vi "LWXPS_CPUCoreAndBoardSupplyVoltagesGet.vi"(1 "XPS Reference IN":refnum<k24>, 4 "LabVIEW error IN":errorcluster) -> (8 "XPS Reference OUT":refnum<k24>, 9 "LabVIEW error OUT":errorcluster, 10 "Returned error code":i32, 11 "XPS Error String":string, 12 "Voltage CPU Core":dbl, 13 "Supply Voltage 5VSB":dbl, 14 "Supply Voltage 1P 5V":dbl, 15 "Supply Voltage 3P 3V":dbl, 16 "Supply Voltage 5V":dbl, 17 "Supply Voltage 12V":dbl, 18 "Supply Voltage M 12V":dbl, 19 "Supply Voltage M 5V":dbl)   [LabVIEW 2014]
uses:
  D:/XPSQ8_LabView_Library/Development/Source/Dll/Newport.XPS.CommandInterface.dll
  Dll/Newport.XPS.CommandInterface.dll
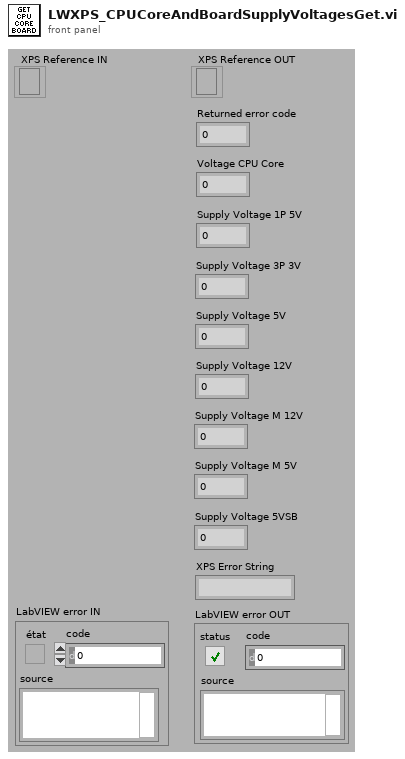
[diagram p1: front panel]
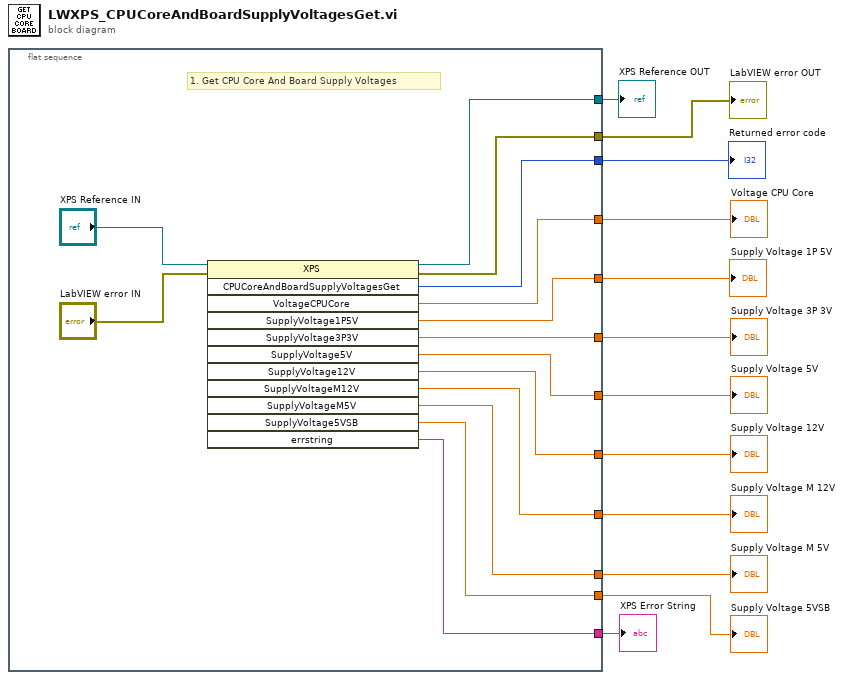
[diagram p0: block diagram]
diagram:
  n1 = flat-sequence {
    tunnel: [w22] -> w12
    tunnel: [w26] -> w1
    tunnel: [w23] -> w11
    tunnel: [w14] -> w9
    tunnel: [w18] -> w10
    tunnel: [w21] -> w8
    tunnel: [w20] -> w7
    tunnel: [w13] -> w6
    tunnel: [w19] -> w5
    tunnel: [w17] -> w4
    tunnel: [w16] -> w3
    tunnel: [w15] -> w2
    frame #0 {
      # "1. Get CPU Core And Board Supply Voltages"
      n2 = invoke class="XPS" method="CPUCoreAndBoardSupplyVoltagesGet"(reference="XPS Reference IN", error in="LabVIEW error IN") -> (reference out=w22:refnum<k24>, error out=w26:errorcluster, "CPUCoreAndBoardSupplyVoltagesGet"=w23:i32, "VoltageCPUCore"=w18:dbl, "SupplyVoltage1P5V"=w14:dbl, "SupplyVoltage3P3V"=w21:dbl, "SupplyVoltage5V"=w20:dbl, "SupplyVoltage12V"=w13:dbl, "SupplyVoltageM12V"=w19:dbl, "SupplyVoltageM5V"=w17:dbl, "SupplyVoltage5VSB"=w16:dbl, "errstring"=w15:string)  [unwired: 10 in]
    }
  }
  "XPS Reference OUT" <- w12
  "LabVIEW error OUT" <- w1
  "Returned error code" <- w11
  "Voltage CPU Core" <- w10
  "Supply Voltage 1P 5V" <- w9
  "Supply Voltage 3P 3V" <- w8
  "Supply Voltage 5V" <- w7
  "Supply Voltage 12V" <- w6
  "Supply Voltage M 12V" <- w5
  "Supply Voltage M 5V" <- w4
  "Supply Voltage 5VSB" <- w3
  "XPS Error String" <- w2
